vi "slink acquire aalhad old code modified.vi"(8 "error in (no error)":errorcluster, 9 "Channel in":T1, 10 "Channel 1":T1, 11 "VISA Refnum in":refnum<visa-resource-name>) -> (0 "error out":errorcluster, 1 "Channel 1 value":dbl, 2 "Channel 2 value":dbl, 3 "VISA Refnum out":refnum<visa-resource-name>)   [LabVIEW 2020, in "Gentec SlinkUSB.lvclass"]
uses:
  Gentec SlinkUSB.lvclass
  shared/OnOffTypeDef.ctl
  Serial Commands Slink.ctl
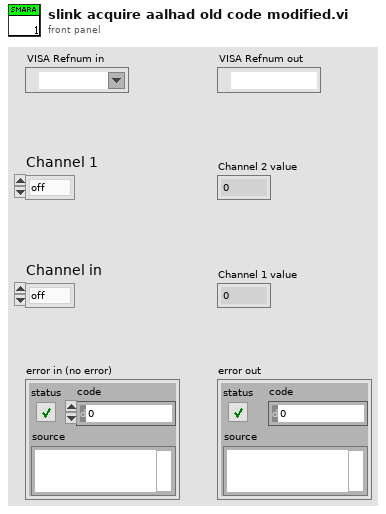
[diagram p1: front panel]
types:
  T1 = typedef "OnOffTypeDef.ctl" = enum16{"off", "on"}
  T2 = typedef "Serial Commands Slink.ctl" = i32
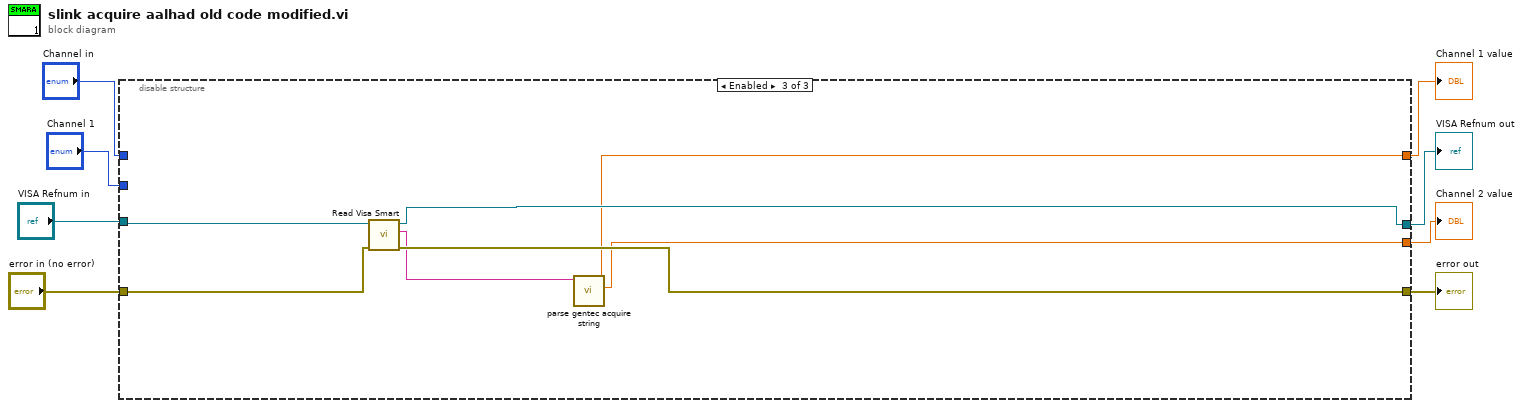
[diagram p0: block diagram]
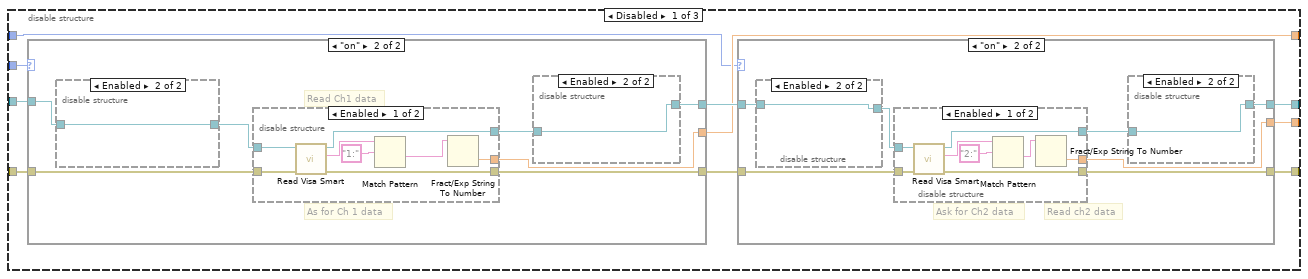
[diagram p2: hidden frame]
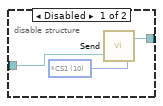
[diagram p4: hidden frame]
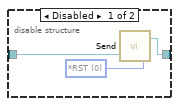
[diagram p5: hidden frame]
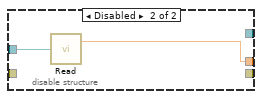
[diagram p6: hidden frame]
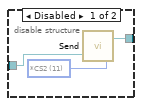
[diagram p8: hidden frame]
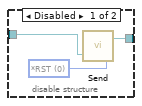
[diagram p9: hidden frame]
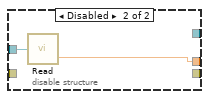
[diagram p10: hidden frame]
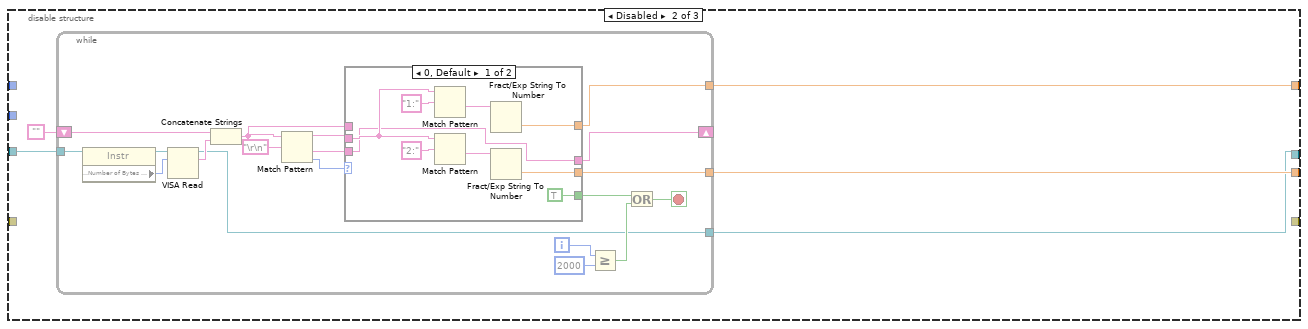
[diagram p11: hidden frame]
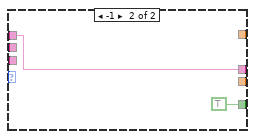
[diagram p12: hidden frame]
diagram:
  n1 = disable-structure shown="Enabled" {
    disable-tunnel: "error in (no error)" -> [w18 _ w112]
    disable-tunnel: [w15 _ w111] -> w2
    disable-tunnel: [w14 w73 w113] -> w3
    disable-tunnel: [w13 w76 w109] -> w4
    disable-tunnel: [w12 w75 w108] -> w5
    disable-tunnel: "Channel 1" -> [w11 _ _]
    disable-tunnel: "Channel in" -> [w10 _ _]
    disable-tunnel: "VISA Refnum in" -> [w9 w74 w114]
    frame Disabled {
      n2 = case shown="\"on\"" w11 {
        tunnel: w9 -> [w20 w21]
        tunnel: w18 -> [w19 w26]
        tunnel: [w20 w22] -> w17
        tunnel: [w19 w25] -> w16
        tunnel: [_ w24] -> w13
        frame "off", Default {
        }
        frame "on" {
          # "Read Ch1 data"
          # "As for Ch 1 data"
          n3 = disable-structure shown="Enabled" {
            disable-tunnel: [w33 w35] -> w27
            disable-tunnel: w21 -> [w32 w35]
            frame Disabled {
              w34 = T2 0 items=["*RST", "*VER", "*CA1", "*CA2", "*SS100", "*SS200", "*SU1", "*SU2", "*SD1", "*SD2", "*CS1", "*CS2", "*AT1", "*AT2", "*AN1", "*AN2", "*PW1", "*PW2", "*TL1", "*TL2", "*ST1", "*ST2", "*ET1", "*ET2", "*EM1", "*EM2", "*SC1", "*SC2", "*VNM", "*CV1", "*CV2"] ("string to write")
              n4 = call "Send.vi"("string to write"=w34, "port number"=w32) -> ("port out"=w33:refnum<visa-resource-name>)  [unwired: 1 in]
            }
            frame Enabled {
            }
          }
          n5 = disable-structure shown="Enabled" {
            disable-tunnel: w27 -> [w43 w45]
            disable-tunnel: w26 -> [w42 _]
            disable-tunnel: [w41 w44] -> w24
            disable-tunnel: [w40 _] -> w23
            disable-tunnel: [w39 _] -> w25
            frame Enabled {
              n6 = call "Read Visa Smart.vi"("error in (no error)"=w42, "VISA Refnum in"=w43) -> ("error out"=w39:errorcluster, "String"=w37:string, "VISA Refnum out"=w40:refnum<visa-resource-name>)  [unwired: 7 in]
              n7 = Match Pattern(string=w37, regular expression="1:") -> (after substring=w36:string)  [unwired: 1 in, 3 out]
              n8 = Fract/Exp String To Number(string=w36) -> (number=w41:dbl)  [unwired: 3 in, 1 out]
            }
            frame Disabled {
              n9 = call "Read.vi"("Com Port"=w45) -> ("Ch 1 out"=w44:dbl)  [unwired: 2 in, 1 out]
            }
          }
          n10 = disable-structure shown="Enabled" {
            disable-tunnel: w23 -> [w29 w31]
            disable-tunnel: [w28 w31] -> w22
            frame Disabled {
              w30 = 10 items=["*RST", "*VER", "*CA1", "*CA2", "*SS100", "*SS200", "*SU1", "*SU2", "*SD1", "*SD2", "*CS1", "*CS2", "*AT1", "*AT2", "*AN1", "*AN2", "*PW1", "*PW2", "*TL1", "*TL2", "*ST1", "*ST2", "*ET1", "*ET2", "*EM1", "*EM2", "*SC1", "*SC2"] ("string to write")
              n11 = call "Send.vi"("string to write"=w30, "port number"=w29) -> ("port out"=w28:refnum<visa-resource-name>)  [unwired: 1 in]
            }
            frame Enabled {
            }
          }
        }
      }
      n12 = case shown="\"on\"" w10 {
        tunnel: w17 -> [w47 w48]
        tunnel: w16 -> [w46 w54]
        tunnel: [w46 w53] -> w15
        tunnel: [w47 w49] -> w14
        tunnel: [_ w52] -> w12
        frame "off", Default {
        }
        frame "on" {
          # "Read ch2 data"
          # "Ask for Ch2 data"
          n13 = disable-structure shown="Enabled" {
            disable-tunnel: [w60 w62] -> w51
            disable-tunnel: w48 -> [w59 w62]
            frame Disabled {
              w61 = T2 0 items=["*RST", "*VER", "*CA1", "*CA2", "*SS100", "*SS200", "*SU1", "*SU2", "*SD1", "*SD2", "*CS1", "*CS2", "*AT1", "*AT2", "*AN1", "*AN2", "*PW1", "*PW2", "*TL1", "*TL2", "*ST1", "*ST2", "*ET1", "*ET2", "*EM1", "*EM2", "*SC1", "*SC2", "*VNM", "*CV1", "*CV2"] ("string to write")
              n14 = call "Send.vi"("string to write"=w61, "port number"=w59) -> ("port out"=w60:refnum<visa-resource-name>)  [unwired: 1 in]
            }
            frame Enabled {
            }
          }
          n15 = disable-structure shown="Enabled" {
            disable-tunnel: w51 -> [w70 w72]
            disable-tunnel: w54 -> [w69 _]
            disable-tunnel: [w68 _] -> w53
            disable-tunnel: [w67 _] -> w50
            disable-tunnel: [w66 w71] -> w52
            frame Enabled {
              n16 = call "Read Visa Smart.vi"("error in (no error)"=w69, "VISA Refnum in"=w70) -> ("error out"=w68:errorcluster, "String"=w64:string, "VISA Refnum out"=w67:refnum<visa-resource-name>)  [unwired: 7 in]
              n17 = Match Pattern(string=w64, regular expression="2:") -> (after substring=w63:string)  [unwired: 1 in, 3 out]
              n18 = Fract/Exp String To Number(string=w63) -> (number=w66:dbl)  [unwired: 3 in, 1 out]
            }
            frame Disabled {
              n19 = call "Read.vi"("Com Port"=w72) -> ("Ch 2 out"=w71:dbl)  [unwired: 2 in, 1 out]
            }
          }
          n20 = disable-structure shown="Enabled" {
            disable-tunnel: w50 -> [w56 w58]
            disable-tunnel: [w55 w58] -> w49
            frame Disabled {
              w57 = 11 items=["*RST", "*VER", "*CA1", "*CA2", "*SS100", "*SS200", "*SU1", "*SU2", "*SD1", "*SD2", "*CS1", "*CS2", "*AT1", "*AT2", "*AN1", "*AN2", "*PW1", "*PW2", "*TL1", "*TL2", "*ST1", "*ST2", "*ET1", "*ET2", "*EM1", "*EM2", "*SC1", "*SC2"] ("string to write")
              n21 = call "Send.vi"("string to write"=w57, "port number"=w56) -> ("port out"=w55:refnum<visa-resource-name>)  [unwired: 1 in]
            }
            frame Enabled {
            }
          }
        }
      }
    }
    frame Disabled {
      n22 = while {
        shift-right: [w94] -> _
        shift-left: "" -> [w91]
        tunnel: w74 -> [w89]
        tunnel: [w80] -> w76
        tunnel: [w79] -> w75
        tunnel: [w78] -> w73
        i -> [w83]
        stop <- w84 stop-if-true
        n23 = property class="Instr"(reference=w89) -> (reference out=w88:refnum<visa-resource-name>, "Serial Settings:Number of Bytes at Serial Port"=w87:u32)  [unwired: 1 in, 1 out]
        n24 = VISA Read(VISA resource name=w88, byte count=w87) -> (VISA resource name out=w78:refnum<visa-resource-name>, read buffer=w81:string)  [unwired: 1 in, 2 out]
        n25 = Concatenate Strings(w91, w81) -> (w95:string)
        n26 = Match Pattern(string=w95, regular expression="\r\n") -> (before substring=w92:string, after substring=w93:string, offset past match=w96:i32)  [unwired: 1 in, 1 out]
        n27 = case shown="0, Default" w96 {
          tunnel: [w99 w107] -> w94
          tunnel: w95 -> [_ w107]
          tunnel: w93 -> [w99 _]
          tunnel: w92 -> [w102 _]
          tunnel: [TRUE ("x") TRUE ("x")] -> w85
          tunnel: [w98 _] -> w80
          tunnel: [w97 _] -> w79
          frame 0, Default {
            n28 = Match Pattern(string=w102, regular expression="1:") -> (after substring=w100:string)  [unwired: 1 in, 3 out]
            n29 = Match Pattern(string=w102, regular expression="2:") -> (after substring=w101:string)  [unwired: 1 in, 3 out]
            n30 = Fract/Exp String To Number(string=w100) -> (number=w98:dbl)  [unwired: 3 in, 1 out]
            n31 = Fract/Exp String To Number(string=w101) -> (number=w97:dbl)  [unwired: 3 in, 1 out]
          }
          frame -1 {
          }
        }
        n32 = Greater Or Equal?(x=w83, y=i16 2000 ("x")) -> (x >= y?=w86:bool)
        n33 = Or(x=w85, y=w86) -> (x .or. y?=w84:bool)
      }
    }
    frame Enabled {
      n34 = call "Read Visa Smart.vi"("error in (no error)"=w112, "VISA Refnum in"=w114) -> ("error out"=w111:errorcluster, "String"=w110:string, "VISA Refnum out"=w113:refnum<visa-resource-name>)  [unwired: 7 in]
      n35 = call "parse gentec acquire string.vi"("Acquisition String"=w110) -> ("Channel 2 value"=w108:dbl, "Channel 1 value"=w109:dbl)  [unwired: 9 in]
    }
  }
  "Channel 2 value" <- w5
  "Channel 1 value" <- w4
  "VISA Refnum out" <- w3
  "error out" <- w2
